vi "MALT XmlNodeReadValue Str.vi"(8 "error in":errorcluster, 10 "XPath":string, 11 "XML File Path":path) -> (0 "error out":errorcluster, 3 "value":string)   [LabVIEW 2018, in "AltonTech MALT200817.lvlib"]
uses:
  AltonTech MALT200817.lvlib
  <vilib>/xml/Close Reference(Node).vi
  <vilib>/xml/NI_XML.lvlib
  <resource>/objmgr/DOMUserDefRef.rc
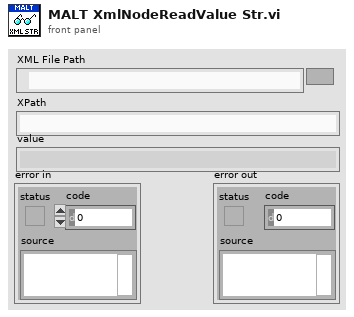
[diagram p1: front panel]
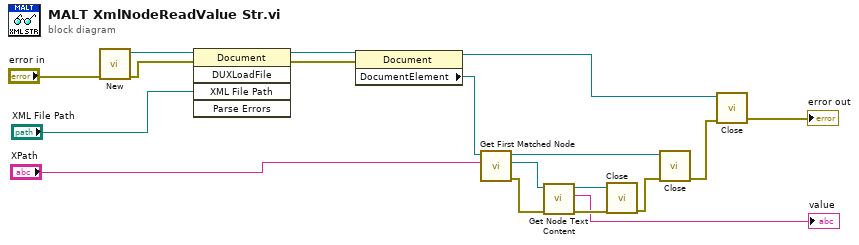
[diagram p0: block diagram]
diagram:
  n1 = call <vilib>:"New.vi"("error in (no error)"="error in") -> ("error out"=w16:errorcluster, "DOM document out"=w18:refnum<k20>)  [unwired: 7 in]
  n2 = invoke class="Document" method="DUXLoadFile"(reference=w18, error in=w16, "XML File Path"="XML File Path") -> (reference out=w14:refnum<k20>, error out=w13:errorcluster)  [unwired: 2 in, 3 out]
  n3 = property class="Document"(reference=w14, error in=w13) -> (reference out=w3:refnum<k20>, "DocumentElement"=w12:refnum<k20>)  [unwired: 1 out]
  n4 = call <vilib>:"Get First Matched Node.vi"("XPath expression"="XPath", "node in"=w12) -> ("error out"=w9:errorcluster, "node result"=w10:refnum<k20>, "node out"=w6:refnum<k20>)  [unwired: 7 in]
  n5 = call <vilib>:"Get Node Text Content.vi"("error in (no error)"=w9, "node in"=w10) -> ("error out"=w8:errorcluster, "node text"=→"value":string, "node out"=w7:refnum<k20>)  [unwired: 7 in]
  n6 = call-poly <vilib>:"Close.vi"("error in (no error)"=w8, "node"=w7) -> ("error out"=w5:errorcluster)  [unwired: 7 in]
  n7 = call-poly <vilib>:"Close.vi"("error in (no error)"=w5, "node"=w6) -> ("error out"=w4:errorcluster)  [unwired: 7 in]
  n8 = call-poly <vilib>:"Close.vi"("error in (no error)"=w4, "node"=w3) -> ("error out"=→"error out":errorcluster)  [unwired: 7 in]
